vi "Get Measurement.vi"(8 "error in (no error)":errorcluster, 9 "Measurement Name":string, 10 "IED Name":string, 11 "SCADA in":refnum<class "SCADA.lvclass">) -> (0 "error out":errorcluster, 3 "SCADA out":refnum<class "SCADA.lvclass">)   [LabVIEW 2015, in "SCADA Core.lvlib" / "SCADA.lvclass"]
uses:
  SCADA.lvclass
  <vilib>/ActorFramework/Actor/Actor.lvclass/Actor.ctl
  SCADA.lvclass/SCADA.ctl
  SCADA Abstract Messages/IED Measurement Status Msg/IED Measurement Status.ctl
  <vilib>/NI/Tools/Keyed Array/Map String.vi
  <vilib>/NI/Tools/String/Get Case Matching.vi
  <vilib>/NI/Tools/Keyed Array/Tools_KeyedArray.lvlib
  <vilib>/ActorFramework/Actor/Actor.lvclass
  SCADA Abstract Messages/IED Measurement Status Msg/IED Measurement Status Msg.lvclass
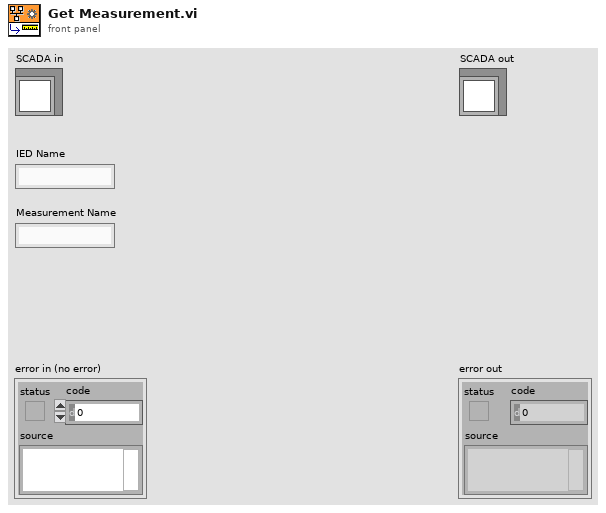
[diagram p1: front panel]
types:
  T1 = typedef "SCADA Core.lvlib/IED Measurement Status Msg.lvclass/IED Measurement Status.ctl" = enum16{"Single Success", "Single Failure", "Multiple Success", "Multiple Failure"}
  T2 = typedef "Tools_KeyedArray.lvlib/KeyedArray.ctl" = cluster{"keys":string[], "values":string[]}
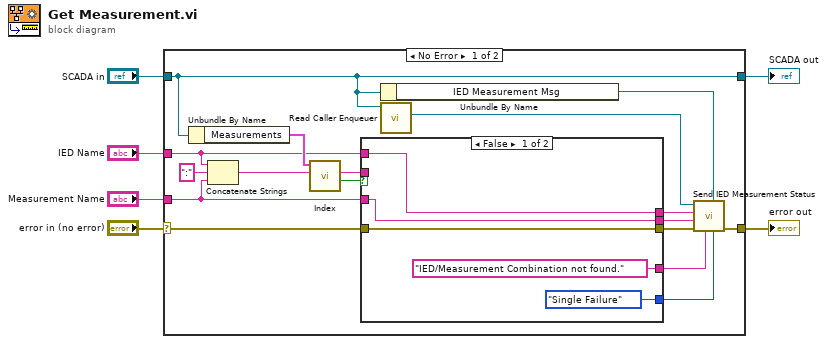
[diagram p0: block diagram]
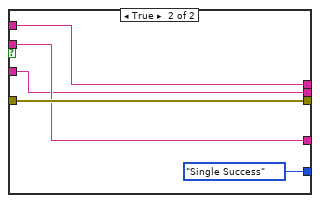
[diagram p2: hidden frame]
diagram:
  n1 = case shown="No Error" "error in (no error)" {
    selector: "error in (no error)" -> [w19 w35]
    tunnel: [w11 w35] -> w5
    tunnel: [w15 w34] -> w3
    tunnel: "SCADA in" -> [w15 w34]
    tunnel: "IED Name" -> [w17 _]
    tunnel: "Measurement Name" -> [w16 _]
    frame No Error {
      n2 = Unbundle By Name(w15) -> ("Measurements"=w22:T2)
      n3 = Concatenate Strings(w17, ":" ("string"), w16) -> (w21:string)
      n4 = call <vilib>:"Index.vi"("key"=w21, "array in"=w22) -> ("valid key"=w20:bool, "value"=w18:string)  [unwired: 3 in, 1 out]
      n5 = case shown="False" w20 {
        tunnel: w19 -> [w28 w33]
        tunnel: w18 -> [_ w31]
        tunnel: w17 -> [w27 w30]
        tunnel: w16 -> [w26 w29]
        tunnel: [w28 w33] -> w12
        tunnel: [IED_Measurement_Status."Single Failure" ("Status") IED_Measurement_Status."Single Success" ("Status")] -> w10
        tunnel: ["IED/Measurement Combination not found." ("value") w31] -> w9
        tunnel: [w27 w30] -> w8
        tunnel: [w26 w29] -> w7
        frame False {
        }
        frame True {
        }
      }
      n6 = Unbundle By Name(w15) -> ("IED Measurement Msg"=w14:refnum<class "IED Measurement Status Msg.lvclass">)
      n7 = call <vilib>:"Read Caller Enqueuer.vi"("Actor"=w15) -> ("Caller Enqueuer"=w13:refnum<class "Message Enqueuer.lvclass">)  [unwired: 10 in]
      n8 = call "Send IED Measurement Status.vi"("Status"=w10, "IED Measurement Msg"=w14, "Value/error"=w9, "error in (no error)"=w12, "Measurement Name"=w7, "IED Name"=w8, "Message Enqueuer in"=w13) -> ("error out"=w11:errorcluster)  [unwired: 3 in, 1 out]
    }
    frame Error {
    }
  }
  "error out" <- w5
  "SCADA out" <- w3
